vi "split string.vi"(2 "Index i":i32=10, 7 "String":string) -> (6 "out 1 (0 bis i-1)":string, 10 "out 2 (i bis n)":string)   [LabVIEW 2010, in "util.lvlib"]
uses:
  util.lvlib
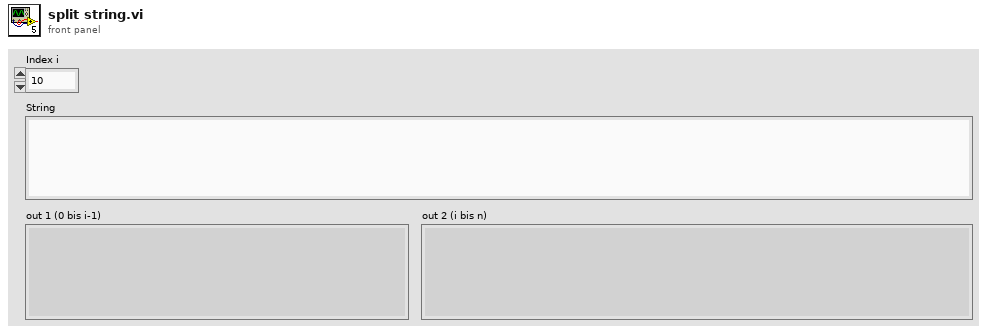
[diagram p1: front panel]
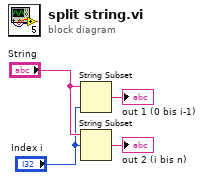
[diagram p0: block diagram]
diagram:
  n1 = String Subset(string="String", length (rest)="Index i") -> (substring=→"out 1 (0 bis i-1)":string)  [unwired: 1 in]
  n2 = String Subset(string="String", offset (0)="Index i") -> (substring=→"out 2 (i bis n)":string)  [unwired: 1 in]
